vi "Close Visa Array.vi"(8 "error in (no error)":errorcluster, 11 "Com in":refnum<visa-resource-name>[](array[refnum])) -> (0 "error out":errorcluster)   [LabVIEW 2019]
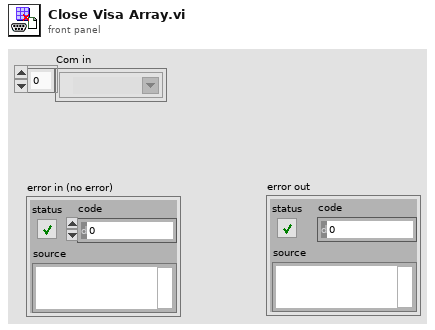
[diagram p1: front panel]
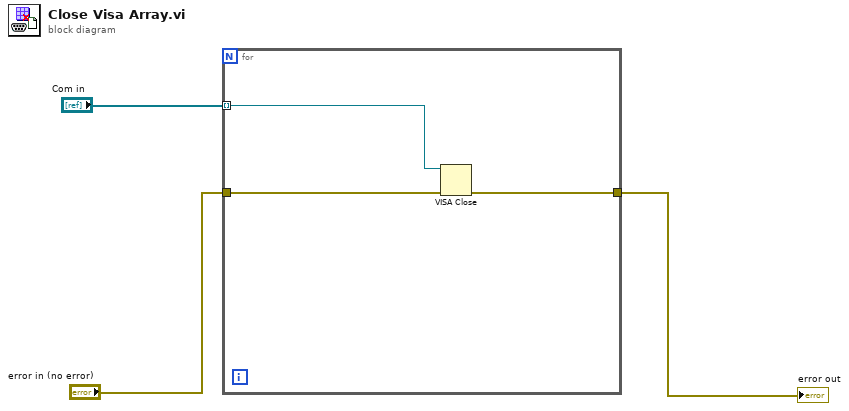
[diagram p0: block diagram]
diagram:
  n1 = for {
    tunnel: "Com in" -> [w6] mode=indexing
    tunnel: [w5] -> w1
    tunnel: "error in (no error)" -> [w4]
    n2 = VISA Close(VISA resource name=w6, error in (no error)=w4) -> (error out=w5:errorcluster)
  }
  "error out" <- w1
